vi "math_ua.vi"(0 "x":dbl[](array[numeric]) format="%0.2f") -> (1 "mean(x)":dbl format="%0.2f", 2 "ua(x)":dbl format="%0.2f", 3 "ua(x) [ppm]":dbl format="%0.2f", 4 "std(x)":dbl format="%0.2f")   [LabVIEW 2013, in "varilib.lvlib"]
doc: "Calculates type A uncertainty of vector of numbers."
uses:
  varilib.lvlib
  <vilib>/Analysis/NI_AALBase.lvlib
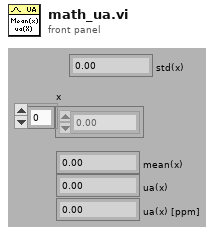
[diagram p1: front panel]
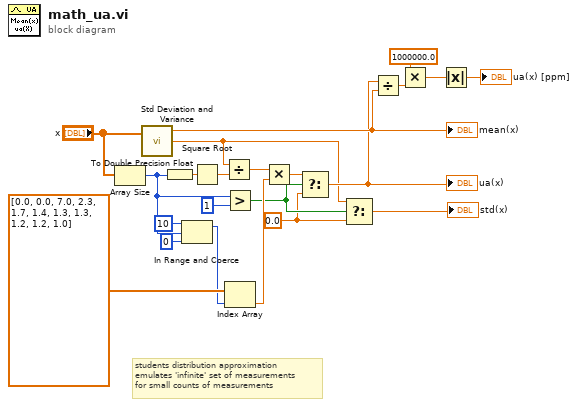
[diagram p0: block diagram]
diagram:
  w1 = 0.0 ("f")
  # "students distribution approximation\nemulates 'infinite' set of measurements\nfor small counts of measurements"
  n1 = Array Size(array="x") -> (size(s)=w8:i32)
  n2 = call <vilib>:"Std Deviation and Variance.vi"("X"="x") -> ("mean"=w13:dbl, "standard deviation"=w3:dbl)  [unwired: 1 in, 1 out]
  "mean(x)" <- w13
  n3 = To Double Precision Float(number=w8) -> (double precision float=w21:dbl)
  n4 = In Range and Coerce(upper limit=10, x=w8, lower limit=0) -> (coerced(x)=w14:i32)  [unwired: 1 out]
  n5 = Square Root(x=w21) -> (sqrt(x)=w20:dbl)
  n6 = Divide(x=w3, y=w20) -> (x/y=w19:dbl)
  n7 = Greater?(x=w8, y=1) -> (0:w2:bool)
  n8 = Index Array(array=dbl[] [0.0, 0.0, 7.0, 2.3, 1.7, 1.4, 1.3, 1.3, 1.2, 1.2, 1.0], index=w14) -> (element=w15:dbl)
  n9 = Multiply(x=w19, y=w15) -> (x*y=w6:dbl)
  n10 = Select(t=w6, s=w2, f=w1) -> (s? t:f=w5:dbl)
  "ua(x)" <- w5
  n11 = Select(t=w3, s=w2, f=w1) -> (s? t:f=→"std(x)":dbl)
  n12 = Divide(x=w5, y=w13) -> (x/y=w12:dbl)
  n13 = Multiply(x=1000000.0, y=w12) -> (x*y=w9:dbl)
  n14 = Absolute Value(x=w9) -> (abs(x)=→"ua(x) [ppm]":dbl)
